vi "stat_f_s3.vi"(5 "Array of Wfm":waveform(i16)[](array[waveform])) -> (1 "Array 2":waveform(i16)[][](array[waveform]))   [LabVIEW 2010]
uses:
  lib/Global 2.vi
  <vilib>/Utility/config.llb/NI_LVConfig.lvlib
panel:
  out "Numeric":i32 caption="Кусков нарезано"
  in  "kD":dbl=1.5
  out "final stops":i32[](array[numeric])
  out "final starts":i32[](array[numeric])
  out "sorted stops":i32[](array[numeric])
  out "sorted starts":i32[](array[numeric])
  # "Удаление пустых промежутков"
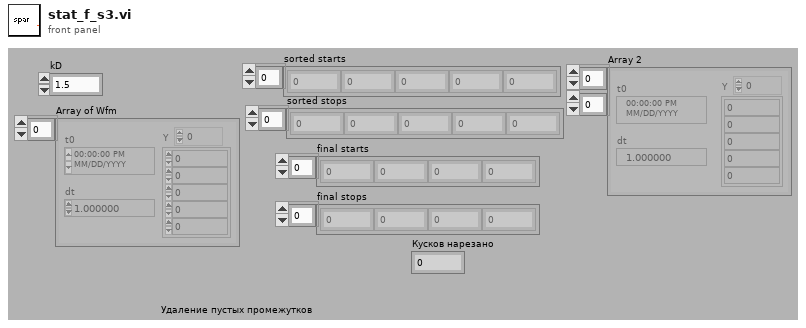
[diagram p1: front panel]
types:
  T1 = typedef "NI_LVConfig.lvlib/Config Data RefNum.ctl" = refnum<k1>
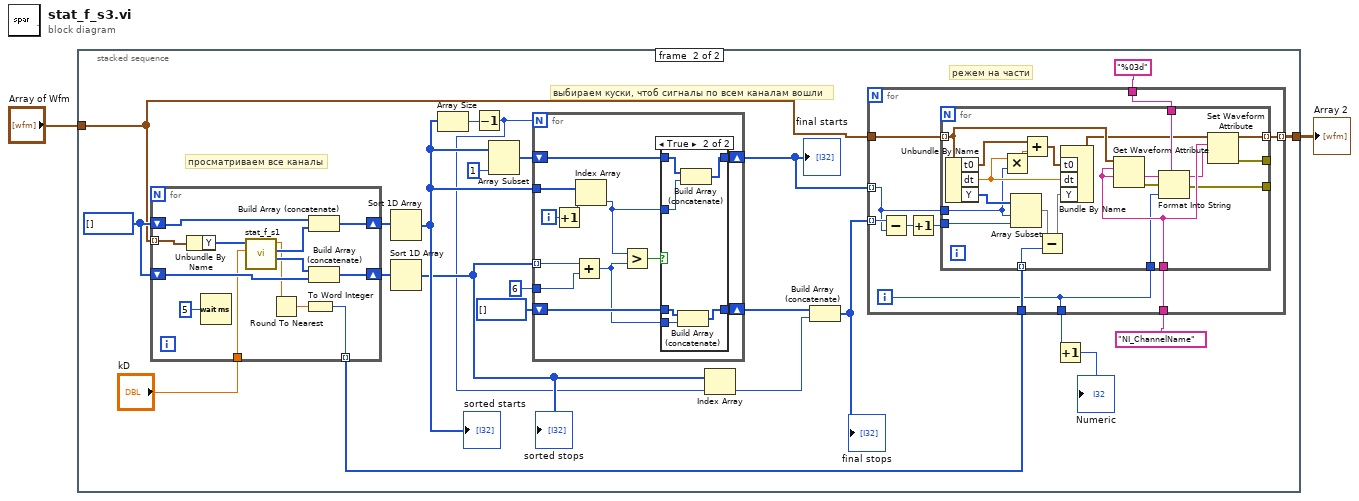
[diagram p0: block diagram]
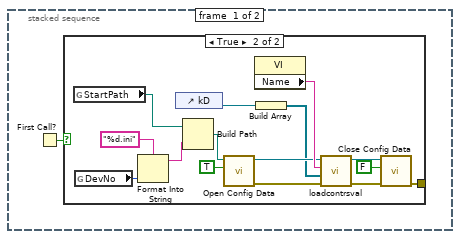
[diagram p2: hidden frame]
diagram:
  n1 = stacked-sequence {
    tunnel: "Array of Wfm" -> [_ w21]
    tunnel: [_ w19] -> w1
    frame #0 {
      n2 = First Call?() -> (First Call?: T/F=w3:bool)
      n3 = case shown="True" w3 {
        tunnel: [_ w17] -> _
        frame False {
        }
        frame True {
          n4 = global read "Global 2.vi" "StartPath"() -> (w4:path)
          n5 = global read "Global 2.vi" "DevNo"() -> (w7:i32)
          n6 = Format Into String(format string="%d.ini", w7) -> (resulting string=w6:string)  [unwired: 2 in, 1 out]
          n7 = control-ref of="kD"() -> (w11:refnum<vi>)
          n8 = Build Path(base path=w4, name or relative path=w6) -> (appended path=w8:path)
          n9 = call <vilib>:"Open Config Data.vi"("create file if necessary (T)"=TRUE, "configuration file path"=w8) -> ("error out"=w16:errorcluster, "refnum"=w13:T1)  [unwired: 7 in, 1 out]
          n10 = property class="VI"() -> ("Name"=w14:string)  [unwired: 2 in, 2 out]
          n11 = Build Array(w11) -> (w10:refnum<vi>[])
          n12 = call "loadcontrsval.vi"("error in"=w16, "Array"=w10, "Section"=w14, "refnum in"=w13) -> ("error out"=w15:errorcluster, "refnum out"=w12:T1)  [unwired: 1 in, 1 out]
          n13 = call <vilib>:"Close Config Data.vi"("error in (no error)"=w15, "write file if changed (T)"=FALSE, "refnum"=w12) -> ("error out"=w17:errorcluster)  [unwired: 7 in, 1 out]
        }
      }
    }
    frame #1 {
      w36 = i32[] []
      # "режем на части"
      # "выбираем куски, чтоб сигналы по всем каналам вошли"
      # "просматриваем все каналы"
      n14 = for {
        tunnel: w21 -> [w104] mode=indexing
        shift-right: [w102] -> w37
        shift-left: w36 -> [w101]
        shift-right: [w99] -> w35
        shift-left: w36 -> [w98]
        tunnel: "kD" -> [w97]
        tunnel: [w94] -> w39 mode=indexing
        n15 = Unbundle By Name(w104) -> ("Y"=w105:i16[])
        n16 = Wait (ms)(milliseconds to wait=u32 5) -> ()  [unwired: 1 out]
        n17 = call "stat_f_s1.vi"("kD"=w97, "Y"=w105) -> ("stops"=w100:i32[], "starts"=w103:i32[], "mean"=w96:dbl)  [unwired: 2 in, 1 out]
        n18 = Round To Nearest(number=w96) -> (nearest integer value=w95:dbl)
        n19 = To Word Integer(number=w95) -> (16bit integer=w94:i16)
        n20 = Build Array (concatenate)(w101, w103) -> (w102:i32[])
        n21 = Build Array (concatenate)(w100, w98) -> (w99:i32[])
      }
      n22 = Sort 1D Array(array=w37) -> (sorted array=w32:i32[])
      "sorted starts" <- w32
      n23 = Sort 1D Array(array=w35) -> (sorted array=w28:i32[])
      "sorted stops" <- w28
      n24 = Array Size(array=w32) -> (size(s)=w31:i32)
      n25 = Decrement(x=w31) -> (x-1=w27:i32)
      n26 = Array Subset(array=w32, length=1) -> (w34:i32[])  [unwired: 1 in]
      n27 = for {
        N: w27 -> [_]
        tunnel: w32 -> [w84]
        tunnel: w28 -> [w77] mode=indexing
        shift-right: [w81] -> w24
        shift-left: w34 -> [w80]
        tunnel: 6 ("length") -> [w78]
        shift-right: [w76] -> w25
        shift-left: i32[] [] -> [w75]
        i -> [w82]
        n28 = Increment(x=w82) -> (x+1=w83:i32)
        n29 = Add(x=w77, y=w78) -> (x+y=w74:i32)
        n30 = Index Array(array=w84, index=w83) -> (element=w73:i32)
        n31 = Greater?(x=w73, y=w74) -> (0:w79:bool)
        n32 = case shown="True" w79 {
          tunnel: w73 -> [_ w92]
          tunnel: [w86 w91] -> w81
          tunnel: w80 -> [w86 w90]
          tunnel: w74 -> [_ w89]
          tunnel: [w85 w88] -> w76
          tunnel: w75 -> [w85 w87]
          frame False {
          }
          frame True {
            n33 = Build Array (concatenate)(w87, w89) -> (w88:i32[])
            n34 = Build Array (concatenate)(w90, w92) -> (w91:i32[])
          }
        }
      }
      "final starts" <- w24
      n35 = Index Array(array=w28, index=w27) -> (element=w26:i32)
      n36 = Build Array (concatenate)(w25, w26) -> (w23:i32[])
      "final stops" <- w23
      n37 = for {
        tunnel: w24 -> [w49] mode=indexing
        tunnel: w23 -> [w51] mode=indexing
        tunnel: w21 -> [w50]
        tunnel: [w47] -> w19 mode=indexing
        tunnel: "NI_ChannelName" ("name") -> [w45]
        tunnel: "%03d" ("format string") -> [w44]
        tunnel: w39 -> [w43]
        tunnel: [w42] -> w40
        i -> [w42]
        n38 = Subtract(x=w51, y=w49) -> (x-y=w48:i32)
        n39 = Increment(x=w48) -> (x+1=w46:i32)
        n40 = for {
          tunnel: w50 -> [w58] mode=indexing
          tunnel: [w55] -> w47 mode=indexing
          tunnel: w49 -> [w59]
          tunnel: w46 -> [w60]
          tunnel: w45 -> [w72]
          tunnel: w42 -> [w71]
          tunnel: w44 -> [w68]
          tunnel: [w66] -> _
          tunnel: [w56] -> _
          tunnel: w43 -> [w53] mode=indexing
          n41 = Unbundle By Name(w58) -> ("t0"=w62:timestamp, "dt"=w64:dbl, "Y"=w61:i16[])
          n42 = Multiply(x=w64, y=w59) -> (x*y=w65:dbl)
          n43 = Array Subset(array=w61, index=w59, length=w60) -> (w54:i16[])
          n44 = Add(x=w62, y=w65) -> (x+y=w63:timestamp)
          n45 = Subtract(x=w54, y=w53) -> (x-y=w52:i16[])
          n46 = Bundle By Name("t0"=w63, "dt"=w64, "Y"=w52) -> (w57:waveform(i16))  [unwired: 1 in]
          n47 = Get Waveform Attribute(5:w72, 6:w72, 7:w58) -> (0:w67:errorcluster, 1:w70:string)  [unwired: 1 in, 2 out]
          n48 = Format Into String(format string=w68, initial string=w70, error in=w67, w71) -> (resulting string=w69:string, error out=w66:errorcluster)
          n49 = Set Waveform Attribute(5:w69, 6:w72, 7:w57) -> (0:w56:errorcluster, 3:w55:waveform(i16))  [unwired: 1 in, 1 out]
        }
      }
      n50 = Increment(x=w40) -> (x+1=→"Numeric":i32)
    }
  }
  "Array 2" <- w1
